vi "Initialize.vi"(0 "VISA resource name":refnum<visa-resource-name>, 1 "Unit Address (1)":u8=1, 5 "ID Query (T: Check)":bool=TRUE, 7 "Reset (T: Reset)":bool=TRUE, 11 "error in (no error)":errorcluster) -> (4 "VISA resource name out":refnum<visa-resource-name>, 15 "error out":errorcluster {"code" format="%.0x"})   [LabVIEW 2010]
doc: "This VI loads the instrument descriptor into the Instr Open VXI VI and returns the instrument ID. You can optionally reset or query the instrument by setting the front panel reset control. You must run this VI before using any of the instrument driver VIs for this instrument.\n\nNotes:\n(1) This instrument driver supports serial communication. If problems are encountered when using serial communication, it is recommended to try using baud rates 9,600 bps or 19,200 bps."
panel:
  # "© 2005 National Instruments.  ALL RIGHTS RESERVED."
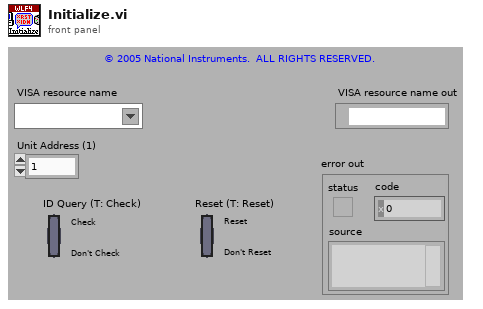
[diagram p1: front panel]
types:
  T1 = cluster{"status":bool, "code":i32, "VI Name":string}
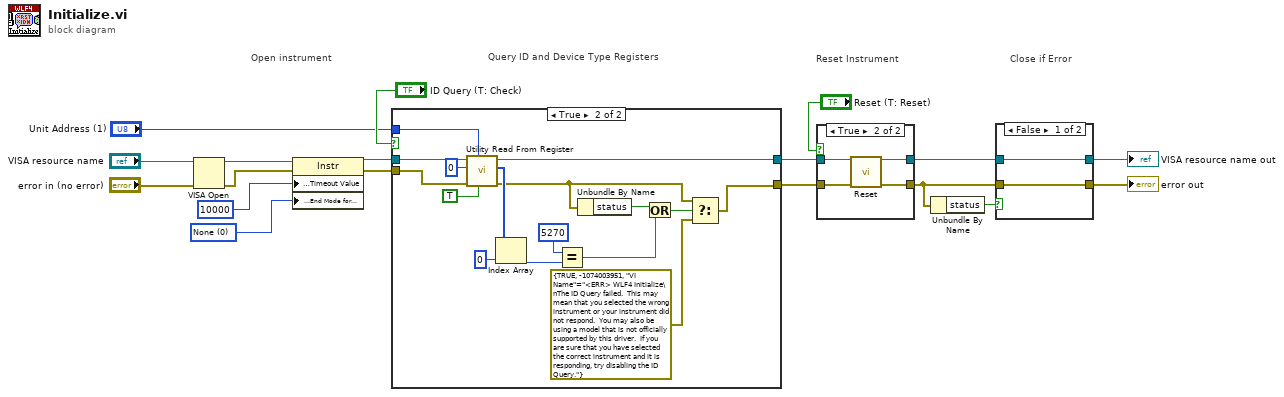
[diagram p0: block diagram]
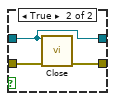
[diagram p2: hidden frame]
diagram:
  w1 = u16 0 items=["None", "LastBit", "TermChar"] ("Serial Settings:Serial End Mode for Reads")
  # "Close if Error"
  # "Query ID and Device Type Registers"
  # "Reset Instrument"
  # "Open instrument"
  n1 = VISA Open(error in (no error)="error in (no error)", VISA resource name="VISA resource name") -> (VISA resource name=w9:refnum<visa-resource-name>, error out=w10:errorcluster)  [unwired: 3 in]
  n2 = property class="Instr"(reference=w9, error in=w10, "General Settings:Timeout Value"=u32 10000, "Serial Settings:End Mode for Reads"=w1) -> (reference out=w4:refnum<visa-resource-name>, error out=w5:errorcluster)
  n3 = case shown="True" "ID Query (T: Check)" {
    tunnel: [w19 w36] -> w18
    tunnel: w5 -> [w19 w28]
    tunnel: w4 -> [w20 w27]
    tunnel: "Unit Address (1)" -> [_ w26]
    tunnel: [w20 w22] -> w2
    frame False {
    }
    frame True {
      n4 = call "Utility Read From Register.vi"("Direct Action?"=TRUE, "Unit Address (1)"=w26, "error in (no error)"=w28, "Register Address (0)"=u16 0 ("Register Address"), "VISA resource name"=w27) -> ("error out"=w29:errorcluster, "Data"=w31:i16[], "VISA resource name out"=w22:refnum<visa-resource-name>)  [unwired: 4 in]
      n5 = Index Array(array=w31, index=0) -> (element=w25:i16)
      n6 = Equal?(x=u16 5270, y=w25) -> (x = y?=w23:bool)
      n7 = Unbundle By Name(w29) -> ("status"=w34:bool)
      n8 = Or(x=w34, y=w23) -> (x .or. y?=w35:bool)
      n9 = Select(t=w29, s=w35, f=cluster{bool, i32, "VI Name":string} {TRUE, -1074003951, "VI Name"="<ERR> WLF4 Initialize\nThe ID Query failed.  This may mean that you selected the wrong instrument or your instrument did not respond.  You may also be using a model that is not officially supported by this driver.  If you are sure that you have selected the correct instrument and it is responding, try disabling the ID Query."}) -> (s? t:f=w36:T1)
    }
  }
  n10 = case shown="True" "Reset (T: Reset)" {
    tunnel: w18 -> [w38 w40]
    tunnel: [w38 w42] -> w11
    tunnel: [w37 w41] -> w12
    tunnel: w2 -> [w37 w39]
    frame False {
    }
    frame True {
      n11 = call "Reset.vi"("VISA resource name"=w39, "error in (no error)"=w40) -> ("VISA resource name out"=w41:refnum<visa-resource-name>, "error out"=w42:errorcluster)  [unwired: 12 in]
    }
  }
  n12 = Unbundle By Name(w11) -> ("status"=w13:bool)
  n13 = case shown="False" w13 {
    tunnel: [w43 w47] -> w14
    tunnel: w12 -> [w44 w46]
    tunnel: [w44 w46] -> w15
    tunnel: w11 -> [w43 w45]
    frame False {
    }
    frame True {
      n14 = call "Close.vi"("VISA resource name"=w46, "error in (no error)"=w45) -> ("error out"=w47:errorcluster)  [unwired: 13 in]
    }
  }
  "VISA resource name out" <- w15
  "error out" <- w14
